vi "SPI Open.vi"(8 "Error In":errorcluster, 10 "SPI Channel (0)":u8, 11 "LINX Resource":T1) -> (0 "Error Out":errorcluster, 3 "LINX Resource":T1)   [LabVIEW 2013, in "LVH-LINX.lvlib"]
doc: "Open the specified SPI channel."
uses:
  <vilib>/LabVIEW Hacker/LINX/LVH-LINX.lvlib
  <vilib>/LabVIEW Hacker/LINX/Private/Type Defs/LINX Ref.ctl
  <vilib>/LabVIEW Hacker/LINX/Private/Type Defs/Platform.ctl
  <vilib>/LabVIEW Hacker/LINX/Private/Type Defs/Interface.ctl
  <vilib>/LabVIEW Hacker/LINX/Private/Device/Type Defs/LINX Device Config.ctl
  <vilib>/LabVIEW Hacker/LINX/Private/Device/Type Defs/TCP Config.ctl
  <vilib>/LabVIEW Hacker/LINX/Private/Type Defs/Device Family.ctl
  <vilib>/LabVIEW Hacker/LINX/Private/Type Defs/Peripheral.ctl
  <vilib>/LabVIEW Hacker/LINX/Private/Type Defs/Channel FGV States.ctl
  <vilib>/LabVIEW Hacker/LINX/Private/Device/Device.lvlib
  <vilib>/LabVIEW Hacker/LINX/Private/myRIO/myRIO.lvlib
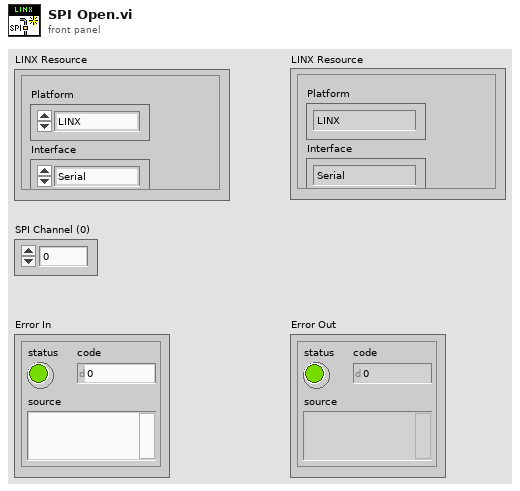
[diagram p1: front panel]
types:
  T1 = typedef "LVH-LINX.lvlib/LINX Ref.ctl" = cluster{"Platform":T2, "Interface":T3, "LINX Device Config":T4}
  T2 = typedef "LVH-LINX.lvlib/Platform.ctl" = enum16{"LINX", "myRIO"}
  T3 = typedef "LVH-LINX.lvlib/Interface.ctl" = enum16{"Serial", "TCP"}
  T4 = typedef "LVH-LINX.lvlib/Device.lvlib/LINX Device Config.ctl" = cluster{"Interface":T3, "COM Port":refnum<visa-resource-name>, "TCP Configuration":T5, "Device Family":T6, "Device ID":u8, "Device Name":string, "TCP Ref":refnum<k5>}
  T5 = typedef "LVH-LINX.lvlib/Device.lvlib/TCP Config.ctl" = cluster{"IP Address":string, "Port":u16}
  T6 = typedef "LVH-LINX.lvlib/Device Family.ctl" = enum8{"National Instruments", "Digilent", "Arduino"}
  T7 = typedef "LVH-LINX.lvlib/Peripheral.ctl" = enum8{"DI", "DO", "AI", "AO", "PWM", "QE", "UART", "I2C", "SPI", "CAN"}
  T8 = typedef "LVH-LINX.lvlib/Channel FGV States.ctl" = enum16{"Initialize", "Get", "Set"}
  T9 = typedef "SPI.lvlib/SPI User Configuration.ctl" = cluster{"Frequency (Hz)":dbl, "Clock Phase":T10, "Clock Polarity":T11, "Data Direction":T12, "Frame Length":T13}
  T10 = typedef "SPI Clock Phase.ctl" = enum8{"Leading", "Trailing"}
  T11 = typedef "SPI Clock Polarity.ctl" = enum8{"Low", "High"}
  T12 = typedef "SPI Data Direction.ctl" = enum8{"Most Significant Bit First", "Least Significant Bit First"}
  T13 = typedef "SPI Frame Length.ctl" = u8
  T14 = typedef "SPI.lvlib/SPI Reference.ctl" = cluster{"myRIO Reference":T15, "SPI Channels Enum":T19, "SPI Configuration":T20}
  T15 = typedef "myRIO Generic Hardware Reference.ctl" = cluster{"myRIO Model":T16, "myRIO Hardware Reference":T17}
  T16 = typedef "Hardware Version Enum.ctl" = enum16{"Unknown", "myRIO-1900", "myRIO-1950"}
  T17 = typedef "myRIO v1.0 Reference.ctl" = cluster{"Generic FPGA Reference":T18, "Allow multiple opens":bool}
  T18 = typedef "Generic FPGA Reference.ctl" = refnum<k20>
  T19 = typedef "SPI Channels Enum.ctl" = enum16{"Not Connected", "A/SPI", "B/SPI"}
  T20 = typedef "SPI.lvlib/SPI Configuration.ctl" = cluster{"Frequency (Hz)":dbl, "Clock Phase":T10, "Clock Polarity":T11, "Data Direction":T12, "Frame Length":T13}
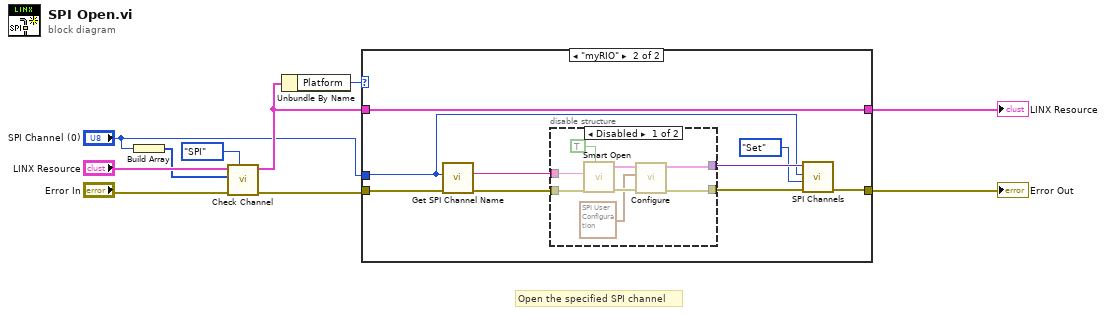
[diagram p0: block diagram]
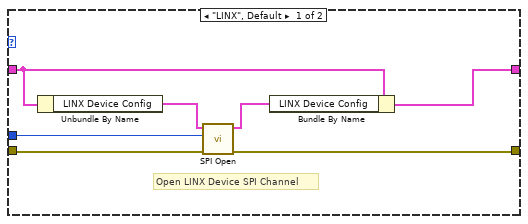
[diagram p2: hidden frame]
diagram:
  # "Open the specified SPI channel"
  n1 = Build Array("SPI Channel (0)") -> (w3:u8[])
  n2 = call <vilib>:"Check Channel.vi"("Peripheral"=Peripheral."SPI", "Error In"="Error In", "Channels"=w3, "LINX Resource"="LINX Resource") -> ("Error Out"=w4:errorcluster, "LINX Resource"=w5:T1)  [unwired: 5 in, 1 out]
  n3 = Unbundle By Name(w5) -> ("Platform"=w10:T2)
  n4 = case shown="\"myRIO\"" w10 {
    tunnel: w4 -> [w14 w25]
    tunnel: w5 -> [w17 w26]
    tunnel: [w15 w22] -> w9
    tunnel: [w16 w26] -> w8
    tunnel: "SPI Channel (0)" -> [w13 w19]
    frame "LINX", Default {
      # "Open LINX Device SPI Channel"
      n5 = Unbundle By Name(w17) -> ("LINX Device Config"=w12:T4)
      n6 = call <vilib>:"SPI Open.vi"("Error In"=w14, "SPI Channel"=w13, "LINX Device Config"=w12) -> ("Error Out"=w15:errorcluster, "LINX Device Config"=w11:T4)  [unwired: 7 in]
      n7 = Bundle By Name(cluster=w17, "LINX Device Config"=w11) -> (w16:T1)
    }
    frame "myRIO" {
      n8 = call <vilib>:"Get SPI Channel Name.vi"("Error In"=w25, "SPI Channel"=w19) -> ("Error Out"=w24:errorcluster, "myRIO SPI Channel"=w21:string)  [unwired: 8 in]
      n9 = disable-structure shown="Disabled" {
        disable-tunnel: w24 -> [w33 _]
        disable-tunnel: [w29 _] -> w23
        disable-tunnel: w21 -> [w32 _]
        disable-tunnel: [w28 _] -> w20
        frame Disabled {
          n10 = call <vilib>:"Smart Open.vi"("Allow multiple opens?"=TRUE, "error in (no error)"=w33, "Channel Name"=w32) -> ("error out"=w30:errorcluster, "SPI Ref Out"=w31:T14)  [unwired: 7 in]
          n11 = call <vilib>:"Configure.vi"("error in (no error)"=w30, "SPI User Configuration"=T9 {"Frequency (Hz)"=0.0, "Clock Phase"=enum."Leading", "Clock Polarity"=enum."Low", "Data Direction"=enum."Most Significant Bit First", "Frame Length"=0}, "SPI Ref In"=w31) -> ("error out"=w29:errorcluster, "SPI Ref Out"=w28:T14)  [unwired: 7 in]
        }
        frame Enabled {
        }
      }
      n12 = call <vilib>:"SPI Channels.vi"("Error In"=w23, "Channel State"=Channel_FGV_States."Set", "Channel Number"=w19, "SPI Channel"=w20) -> ("Error Out"=w22:errorcluster)  [unwired: 6 in, 1 out]
    }
  }
  "Error Out" <- w9
  "LINX Resource" <- w8
